vi "plcm3OpenUnit.vi"(1 "IP Address:port number":string="192.168.1.30:6250", 5 "Serial Number":string, 7 "Use Serial Number":bool, 8 "error in (no error)":errorcluster, 9 "Enumerate USB/Ethernet/ALL":u32(ring)=4294967295 items=["USB"=1, "Ethernet"=2, "ALL"=4294967295], 10 "Connection":bool=TRUE, 11 "Mode":u16(ring) items=["Dialog On Error", "no dialog - CloseUnit and Stop", "no dialog - Continue", "no dialog - Stop"]) -> (0 "error out":errorcluster, 2 "Unit Info":T1, 3 "handle out":i16=16384, 4 "plcm3 Units":string, 6 "serialLth":u32=13)   [LabVIEW 2010]
doc: "This VI manages listing and opens devices with device details."
uses:
  plcm3.dll
panel:
  # "USB"
  # "Ethernet"
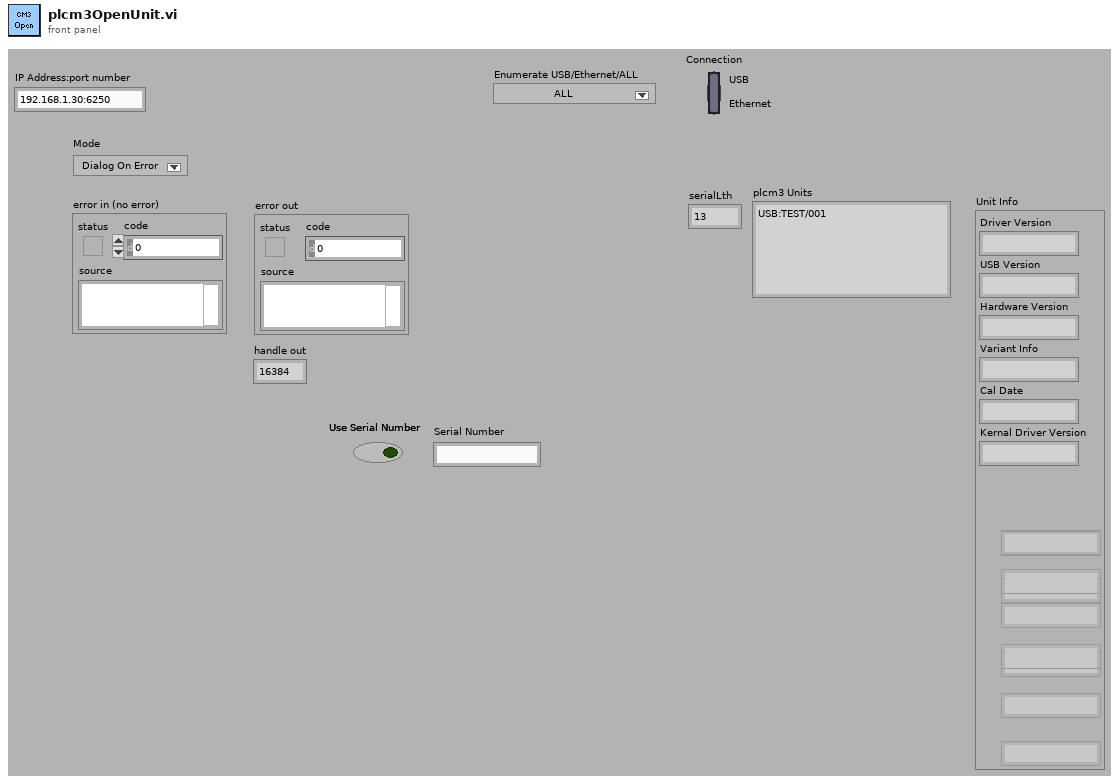
[diagram p1: front panel]
types:
  T1 = cluster{"Driver Version":string, "USB Version":string, "Hardware Version":string, "Variant Info":string, "Cal Date":string, "Kernal Driver Version":string, "NA":string, "NA 2":string, "NA":string, "NA 3":string, "NA 4":string, "NA 5":string, "NA 6":string, "NA 7":string, "NA 8":string}
  T2 = cluster{"status":bool, "code":u32, "source":string}
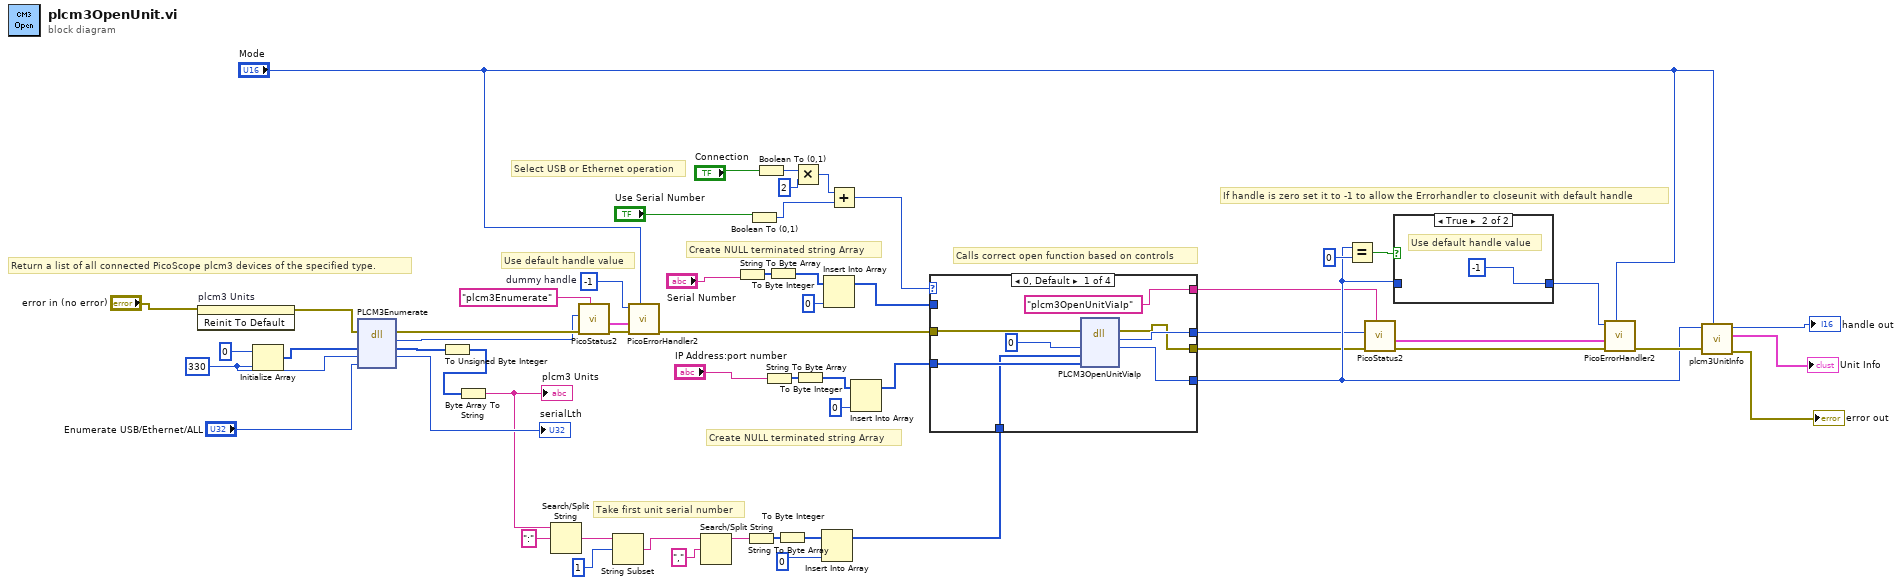
[diagram p0: block diagram]
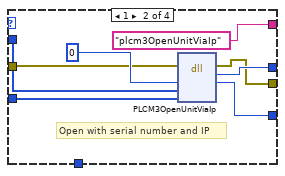
[diagram p3: hidden frame]
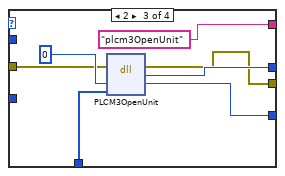
[diagram p4: hidden frame]
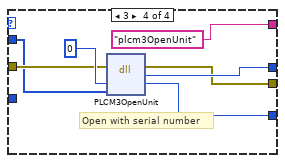
[diagram p5: hidden frame]
diagram:
  w27 = i16 -1  # dummy handle
  w44 = u32 330 ("dimension size")
  # "Take first unit serial number"
  # "If handle is zero set it to -1 to allow the Errorhandler to closeunit with default handle"
  # "Calls correct open function based on controls"
  # "Use default handle value"
  # "Create NULL terminated string Array"
  # "Create NULL terminated string Array"
  # "Return a list of all connected PicoScope plcm3 devices of the specified type."
  # "Select USB or Ethernet operation"
  n1 = invoke on="plcm3 Units" class="Str" method="Reinit To Default"(error in="error in (no error)") -> (error out=w41:errorcluster)  [unwired: 2 in, 2 out]
  n2 = Initialize Array(i8 0 ("U8"), w44) -> (w45:i8[])
  n3 = dll-call lib="plcm3.dll" fn="PLCM3Enumerate"(error in=w41, "details_str"=w45, "length"=w44, "type"="Enumerate USB/Ethernet/ALL") -> (error out=w20:errorcluster, "PICO_STATUS"=w19:u32, "details_str"=w42:i8[], "length"=→"serialLth":u32)  [unwired: 3 in, 1 out]
  n4 = To Unsigned Byte Integer(number=w42) -> (unsigned 8bit integer=w43:u8[])
  n5 = Byte Array To String(unsigned byte array=w43) -> (string=w3:string)
  "plcm3 Units" <- w3
  n6 = Search/Split String(string=w3, search string/char (-)=":") -> (match + rest of string=w5:string)  [unwired: 1 in, 2 out]
  n7 = call "PicoStatus2.vi"("PICO source"="plcm3Enumerate" ("source"), "Error in"=w20, "PICO STATUS"=w19) -> ("error out"=w22:errorcluster, "PICO_STATUS out"=w21:T2)  [unwired: 5 in]
  n8 = String Subset(string=w5, offset (0)=1) -> (substring=w4:string)  [unwired: 1 in]
  n9 = call "PicoErrorHandler2.vi"("Mode"="Mode", "error in (no error)"=w22, "PICO_STATUS in"=w21, "handle In"=w27) -> ("error out"=w28:errorcluster)  [unwired: 7 in]
  n10 = Search/Split String(string=w4, search string/char (-)=",") -> (substring before match=w7:string)  [unwired: 1 in, 2 out]
  n11 = String To Byte Array(string="Serial Number") -> (unsigned byte array=w33:u8[])
  n12 = String To Byte Array(string=w7) -> (unsigned byte array=w10:u8[])
  n13 = Boolean To (0,1)(Boolean="Use Serial Number") -> (0, 1=w54:i16)
  n14 = Boolean To (0,1)(Boolean="Connection") -> (0, 1=w57:i16)
  n15 = String To Byte Array(string="IP Address:port number") -> (unsigned byte array=w38:u8[])
  n16 = To Byte Integer(number=w33) -> (8bit integer=w32:i8[])
  n17 = To Byte Integer(number=w10) -> (8bit integer=w11:i8[])
  n18 = Multiply(x=w57, y=i16 2) -> (x*y=w55:i16)
  n19 = To Byte Integer(number=w38) -> (8bit integer=w37:i8[])
  n20 = Insert Into Array(array=w11, new element=i8 0 ("new element/subarray")) -> (w2:i8[])  [unwired: 1 in]
  n21 = Insert Into Array(array=w32, new element=i8 0 ("new element/subarray")) -> (w29:i8[])  [unwired: 1 in]
  n22 = Add(x=w55, y=w54) -> (x+y=w53:i16)
  n23 = Insert Into Array(array=w37, new element=i8 0 ("new element/subarray")) -> (w34:i8[])  [unwired: 1 in]
  n24 = case shown="0, Default" w53 {
    tunnel: [w66 w73 w81 w88] -> w14
    tunnel: [w65 w72 w79 w86] -> w23
    tunnel: [w64 w71 w80 w87] -> w15
    tunnel: w28 -> [w63 w70 w77 w84]
    tunnel: w29 -> [_ w69 _ w83]
    tunnel: w34 -> [w62 w68 _ _]
    tunnel: ["plcm3OpenUnitViaIp" ("source") "plcm3OpenUnitViaIp" ("source") "plcm3OpenUnit" ("source") "plcm3OpenUnit" ("source")] -> w13
    tunnel: w2 -> [w59 _ w75 _]
    frame 0, Default {
      n25 = dll-call lib="plcm3.dll" fn="PLCM3OpenUnitViaIp"(error in=w63, "handle"=i16 0, "serial"=w59, "IpAddress"=w62) -> (error out=w64:errorcluster, "PICO_STATUS"=w66:u32, "handle"=w65:i16)  [unwired: 4 in, 1 out]
    }
    frame 1 {
      # "Open with serial number and IP"
      n26 = dll-call lib="plcm3.dll" fn="PLCM3OpenUnitViaIp"(error in=w70, "handle"=i16 0, "serial"=w69, "IpAddress"=w68) -> (error out=w71:errorcluster, "PICO_STATUS"=w73:u32, "handle"=w72:i16)  [unwired: 4 in, 1 out]
    }
    frame 2 {
      n27 = dll-call lib="plcm3.dll" fn="PLCM3OpenUnit"(error in=w77, "handle"=i16 0, "serial"=w75) -> (error out=w80:errorcluster, "PICO_STATUS"=w81:u32, "handle"=w79:i16)  [unwired: 3 in, 1 out]
    }
    frame 3 {
      # "Open with serial number"
      n28 = dll-call lib="plcm3.dll" fn="PLCM3OpenUnit"(error in=w84, "handle"=i16 0, "serial"=w83) -> (error out=w87:errorcluster, "PICO_STATUS"=w88:u32, "handle"=w86:i16)  [unwired: 3 in, 1 out]
    }
  }
  n29 = Equal?(x=w23, y=i16 0) -> (x = y?=w24:bool)
  n30 = call "PicoStatus2.vi"("PICO source"=w13, "Error in"=w15, "PICO STATUS"=w14) -> ("error out"=w17:errorcluster, "PICO_STATUS out"=w16:T2)  [unwired: 5 in]
  n31 = case shown="True" w24 {
    tunnel: [w89 i16 -1 ("handle In")] -> w26
    tunnel: w23 -> [w89 _]
    frame False {
    }
    frame True {
      # "Use default handle value"
    }
  }
  n32 = call "PicoErrorHandler2.vi"("Mode"="Mode", "error in (no error)"=w17, "PICO_STATUS in"=w16, "handle In"=w26) -> ("error out"=w39:errorcluster)  [unwired: 7 in]
  n33 = call "plcm3UnitInfo.vi"("Mode"="Mode", "error in (no error)"=w39, "handle in"=w23) -> ("error out"=→"error out":errorcluster, "Unit Info"=→"Unit Info":T1, "handle out"=→"handle out":i16)  [unwired: 6 in]
